vi "Limelight_Differential.vi"() -> (0 "TargetValid":bool, 2 "SteerCommand":dbl(knob)=nan scale=-1.0..1.0, 3 "DriveCommand":dbl(knob)=-0.0 scale=-1.0..1.0)   [LabVIEW 2020]
uses:
  <vilib>/Rock Robotics/Network Tables/NT Read Number.vi
  Framework/Robot Global Data.vi
panel:
  out "Steer & Throtle":dbl[](graph)
  out "ta":dbl(graph)
  out "Tx":dbl(graph)
  out "tv Valid Target":dbl(graph)
  out "MaxDrive":dbl(slide)=0.6824817518248175 min=0.0 max=1.0 step=0.01 scale=0.0..1.0
  out "DriveK":dbl(slide)=0.26277372262773724 min=0.0 max=1.0 step=0.05 scale=0.0..1.0
  out "Limelight Goal Area":dbl(slide)=14.8723 min=0.1 max=25.0 step=0.25 scale=0.0..25.0
  out "AimDeadband":dbl min=0.0 max=10.0 step=0.25
  out "MinSteerCommand":dbl(slide)=0.2717391304347826 min=0.0 max=0.5 step=0.05 scale=0.0..0.5
  out "SteeringK":dbl(slide)=0.025362318840579712 min=0.0 max=0.25 step=0.01 scale=0.0..0.25
  # "0.0253623"
  # "0.271739"
  # "14.8723"
  # "0.262774"
  # "0.682482"
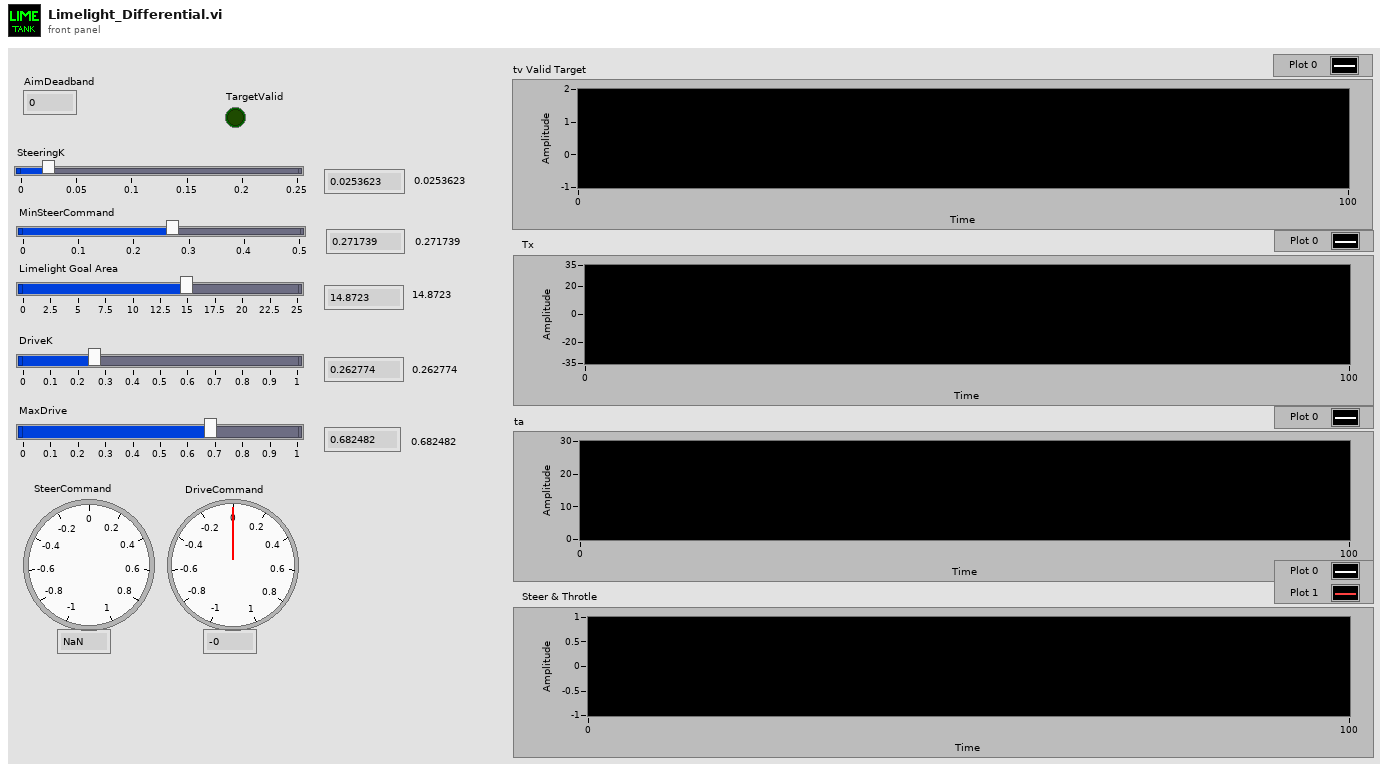
[diagram p1: front panel]
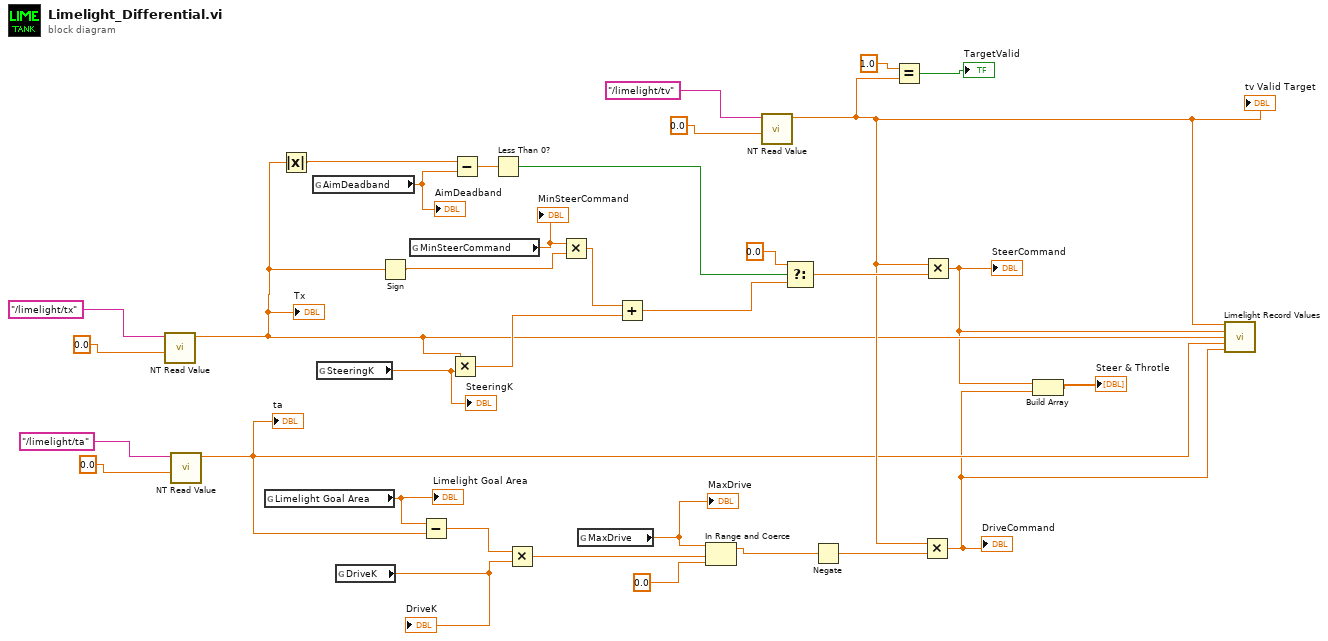
[diagram p0: block diagram]
diagram:
  n1 = call-poly <vilib>:"NT Read Value.vi"("Default Value"=0.0, "Name"="/limelight/tx") -> ("Numeric"=w5:dbl)  [unwired: 8 in, 1 out]
  "Tx" <- w5
  n2 = call-poly <vilib>:"NT Read Value.vi"("Default Value"=0.0, "Name"="/limelight/ta") -> ("Numeric"=w4:dbl)  [unwired: 8 in, 1 out]
  "ta" <- w4
  n3 = global read "Robot Global Data.vi" "Limelight Goal Area"() -> (w9:dbl)
  "Limelight Goal Area" <- w9
  n4 = Absolute Value(x=w5) -> (abs(x)=w31:dbl)
  n5 = global read "Robot Global Data.vi" "AimDeadband"() -> (w12:dbl)
  "AimDeadband" <- w12
  n6 = global read "Robot Global Data.vi" "SteeringK"() -> (w10:dbl)
  "SteeringK" <- w10
  n7 = global read "Robot Global Data.vi" "DriveK"() -> (w7:dbl)
  "DriveK" <- w7
  n8 = Sign(1:w5) -> (0:w21:dbl)
  n9 = global read "Robot Global Data.vi" "MinSteerCommand"() -> (w11:dbl)
  "MinSteerCommand" <- w11
  n10 = Subtract(x=w9, y=w4) -> (x-y=w20:dbl)
  n11 = Multiply(x=w5, y=w10) -> (x*y=w29:dbl)
  n12 = Subtract(x=w31, y=w12) -> (x-y=w32:dbl)
  n13 = Less Than 0?(x=w32) -> (x < 0?=w33:bool)
  n14 = Multiply(x=w20, y=w7) -> (x*y=w19:dbl)
  n15 = Multiply(x=w11, y=w21) -> (x*y=w30:dbl)
  n16 = global read "Robot Global Data.vi" "MaxDrive"() -> (w8:dbl)
  "MaxDrive" <- w8
  n17 = Add(x=w30, y=w29) -> (x+y=w15:dbl)
  n18 = In Range and Coerce(upper limit=w8, x=w19, lower limit=0.0) -> (coerced(x)=w17:dbl)  [unwired: 1 out]
  n19 = call-poly <vilib>:"NT Read Value.vi"("Default Value"=0.0, "Name"="/limelight/tv") -> ("Numeric"=w6:dbl)  [unwired: 8 in, 1 out]
  "tv Valid Target" <- w6
  n20 = Select(t=0.0, s=w33, f=w15) -> (s? t:f=w22:dbl)
  n21 = Negate(x=w17) -> (-x=w16:dbl)
  n22 = Equal?(x=1.0, y=w6) -> (x = y?=→"TargetValid":bool)
  n23 = Multiply(x=w6, y=w16) -> (x*y=w1:dbl)
  "DriveCommand" <- w1
  n24 = Multiply(x=w6, y=w22) -> (x*y=w2:dbl)
  "SteerCommand" <- w2
  n25 = Build Array(w2, w1) -> (→"Steer & Throtle":dbl[])
  n26 = call "Limelight Record Values.vi"("tv"=w6, "Steer"=w2, "tx"=w5, "ta"=w4, "Drive"=w1) -> ()  [unwired: 11 in]
